vi "AP2_photoelectron_image_aquisition.vi"() -> ()   [LabVIEW 2023]
panel:
  in  "Tuning Spline Path":path
  in  "Tab Control 2":enum32{"Image Slice"}(tab)
  out "Image Slice":dbl[](graph)
  in  "Calc R pixel":bool
  in  "Center Y":dbl=555.0
  in  "Center X":dbl=548.0
  in  "Tab Control":T1(tab)
  out "B Counts/5F":dbl
  out "Avg Counts/F":dbl
  out "A Counts":u32
  out "B Counts":u32
  out "Total Counts":u32
  out "A Counts/5F":dbl
  in  "Stop Control":bool
  in  "Save Image Button":bool
  in  "Discard Image Button":bool
  in  "Threshold range":cluster{"Lower value":sgl, "Upper value":sgl}={"Lower value"=6.0, "Upper value"=1024.0}
  in  "Region of interest":i32[](array[numeric])
  in  "Number of buffers":u32
  in  "Frame timeout (ms)":u32=1000
  in  "Update img":bool
  out "FPS":dbl
  out "Processing time / ms":u32
  in  "Frequency Doubled":bool
  out "Current Wavelength":dbl
  in  "Wavelength":dbl
  out "Accumulated Image":i16[][](graph)
  # "Monitoring"
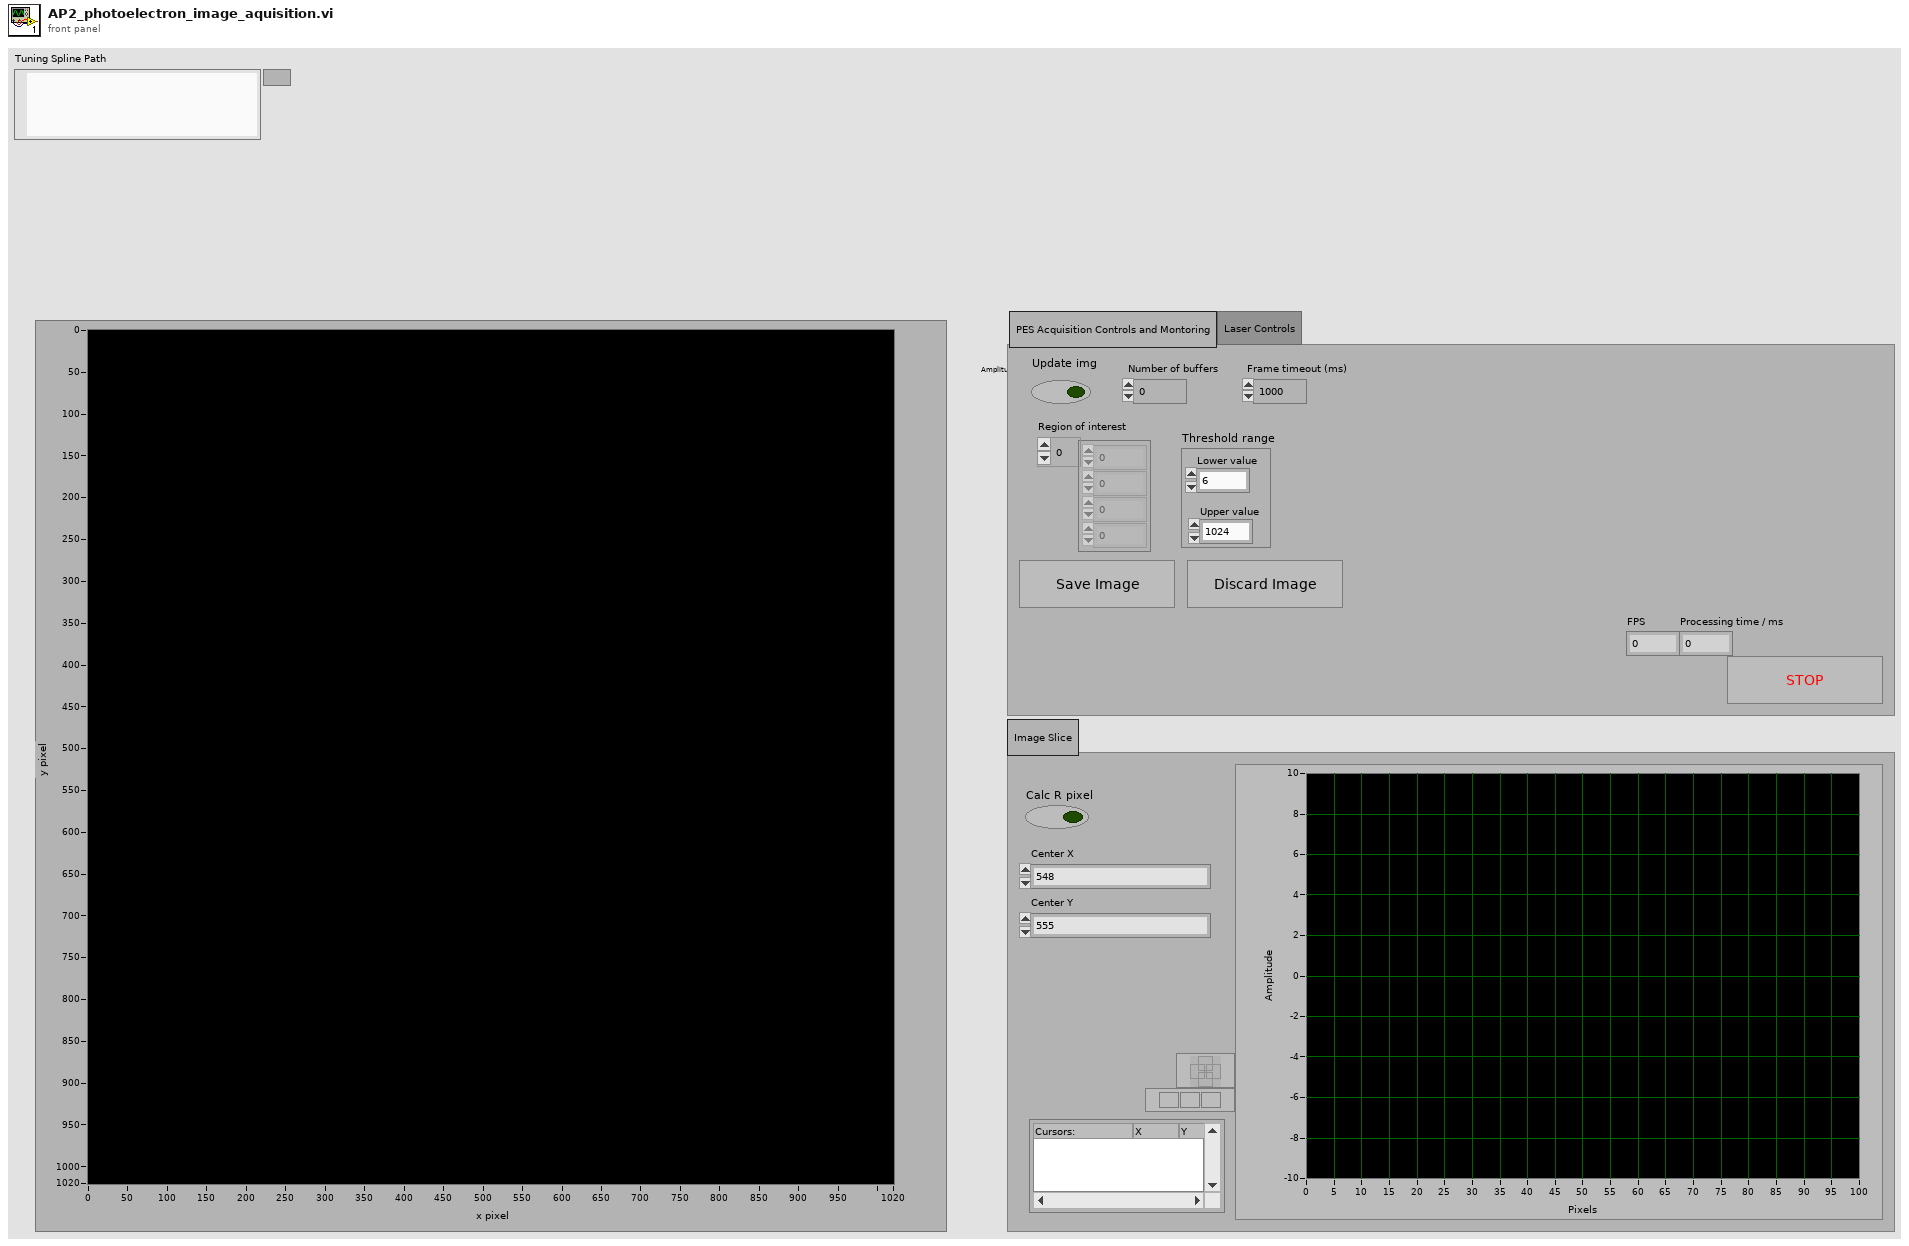
[diagram p1: front panel]
types:
  T1 = enum32{"PES Acquisition Controls and Montoring", "Laser Controls"}
  T2 = cluster{"Region of interest":i32[], "Number of buffers":u32, "Frame timeout (ms)":u32}
  T3 = cluster{"queue out":refnum<queue>, "error out":errorcluster}
  T4 = cluster{"notifier out":refnum<notifier>, "error out":errorcluster}
  T5 = cluster{"i01 data":sgl[][], "i02 data":sgl[][], "Count Buffer Size Out":i32, "Empty Image":i16[][], "Accumulated Image":i16[][], "Corrected Image 1":i16[][], "Corrected Image 2":i16[][], "Total counts":i32, "t_1":i32, "t_2":i32, "t_3":i32, "t_4":i32, "t_5":i32, "t_6":i32, "t_7":i32, "t_8":i32, "t_9":i32, "t_10":i32, "c_1":i32, "c_2":i32, "Region of interest":i32[]}
  T6 = cluster{"Total Counts":u32, "Avg Counts/F":dbl, "B Counts":u32, "A Counts":u32, "A Counts/5F":dbl, "B Counts/5F":dbl}
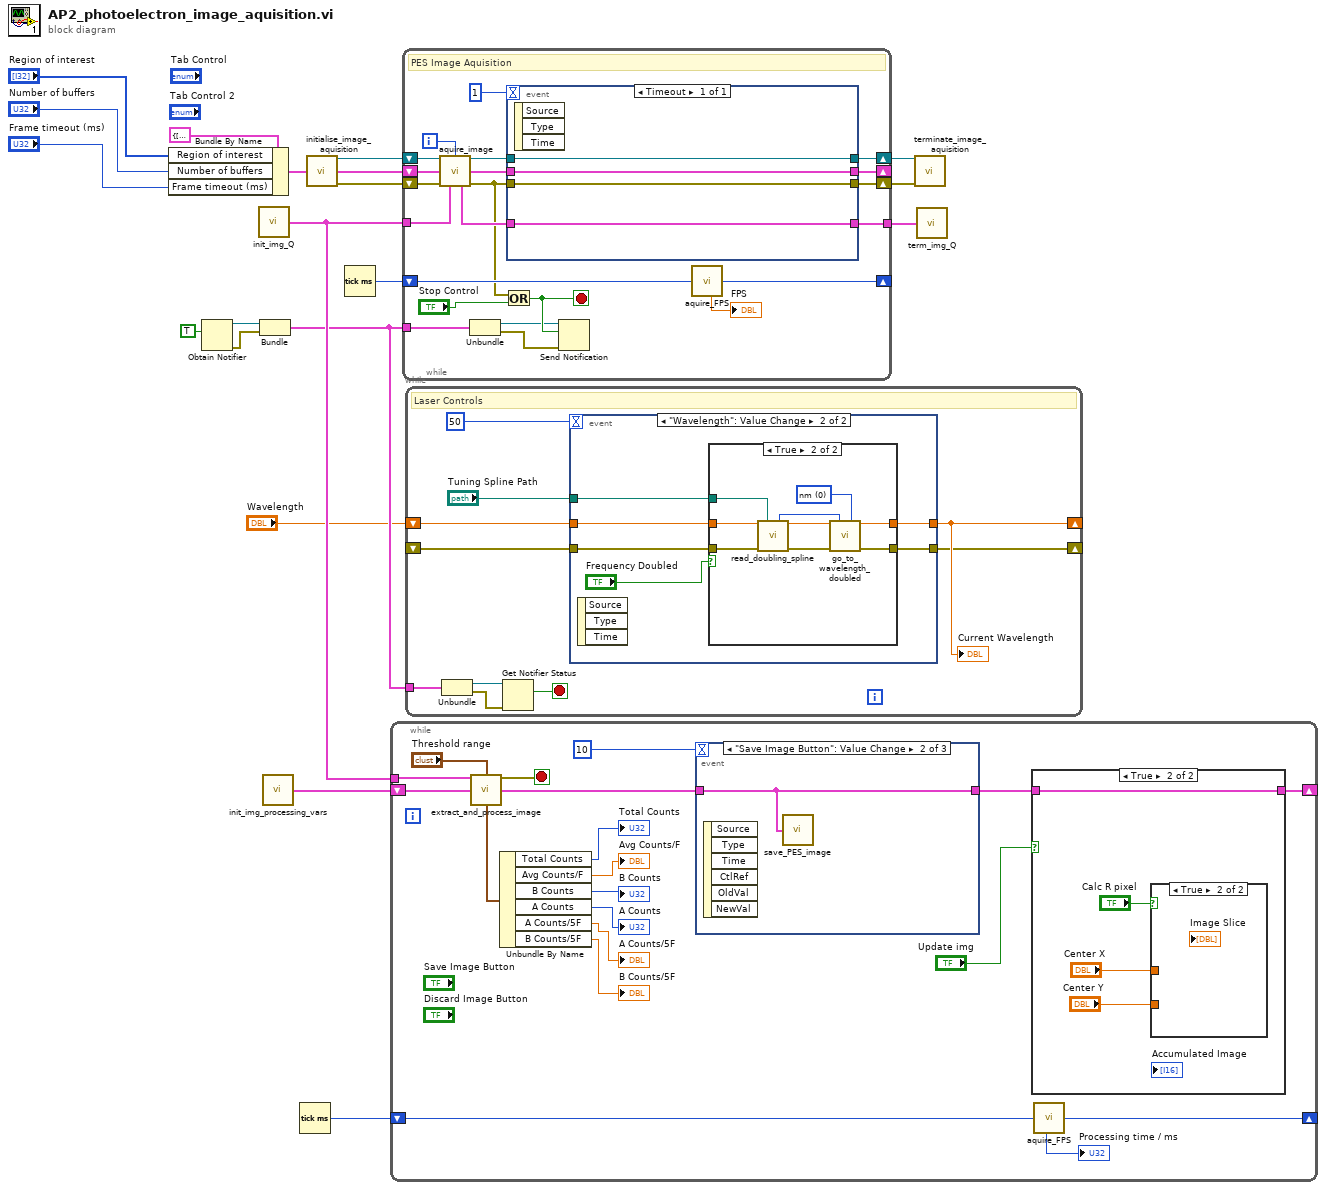
[diagram p0: block diagram]
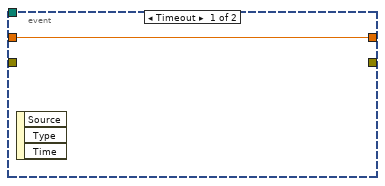
[diagram p2: hidden frame]
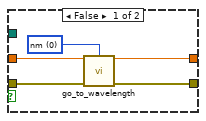
[diagram p3: hidden frame]
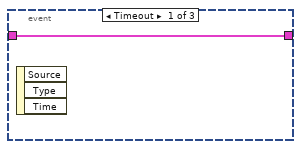
[diagram p4: hidden frame]
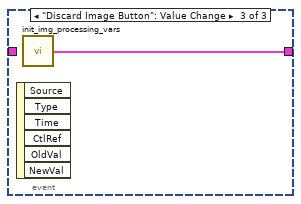
[diagram p5: hidden frame]
diagram:
  n1 = Bundle By Name(cluster=T2 {"Region of interest"=[], "Number of buffers"=0, "Frame timeout (ms)"=1000}, "Region of interest"="Region of interest", "Number of buffers"="Number of buffers", "Frame timeout (ms)"="Frame timeout (ms)") -> (w14:T2)
  n2 = Obtain Notifier(notification data type=TRUE) -> (notifier out=w4:refnum<notifier>, error out=w3:errorcluster)  [unwired: 3 in, 1 out]
  n3 = call "init_img_Q.vi"() -> ("Image Q Out"=w11:T3)  [unwired: 15 in]
  n4 = Bundle("notifier out"=w4, "error out"=w3) -> (w2:T4)  [unwired: 1 in]
  n5 = call "init_img_processing_vars.vi"() -> ("Image Processing Data"=w7:T5)  [unwired: 15 in]
  n6 = Tick Count (ms)() -> (millisecond timer value=w8:u32)
  n7 = call "initialise_image_aquisition.vi"("Imaging Variables In"=w14) -> ("IMAQ Session Out"=w20:refnum<k11>, "Imaging Variables Out"=w13:T2, "error out"=w19:errorcluster)  [unwired: 11 in, 1 out]
  n8 = Tick Count (ms)() -> (millisecond timer value=w6:u32)
  n9 = while {
    tunnel: w11 -> [w36]
    shift-right: [w37] -> _
    shift-left: w8 -> [w38]
    shift-right: [w33] -> _
    shift-left: w7 -> [w34]
    stop <- w35 stop-if-true
    n10 = call "extract_and_process_image.vi"("Image Q In"=w36, "Threshold range"="Threshold range", "Processed Image Data In"=w34) -> ("error out"=w35:errorcluster, "Processed Image Data Out"=w31:T5, "Count data"=w28:T6)  [unwired: 10 in]
    n11 = Unbundle By Name(w28) -> ("Total Counts"=→"Total Counts":u32, "Avg Counts/F"=→"Avg Counts/F":dbl, "B Counts"=→"B Counts":u32, "A Counts"=→"A Counts":u32, "A Counts/5F"=→"A Counts/5F":dbl, "B Counts/5F"=→"B Counts/5F":dbl)
    n12 = event shown="[1] \"Save Image Button\": Value Change" {
      selector: _ -> [_ _ _]
      dyn-events: _ -> [_ _ _]
      timeout: 10 -> [_ _ _]
      tunnel: w31 -> [w40 w41 _]
      tunnel: [w40 w41 w42] -> w29
      event Timeout {
        n13 = event-data() -> ()  [unwired: 1 in, 3 out]
      }
      event "Save Image Button": Value Change {
        n14 = event-data() -> ()  [unwired: 1 in, 6 out]
        n15 = call "save_PES_image.vi"("Processed Image Data In"=w41) -> ()  [unwired: 15 in]
      }
      event "Discard Image Button": Value Change {
        n16 = event-data() -> ()  [unwired: 1 in, 6 out]
        n17 = call "init_img_processing_vars.vi"() -> ("Image Processing Data"=w42:T5)  [unwired: 15 in]
      }
    }
    n18 = case shown="True" "Update img" {
      tunnel: w29 -> [w43 w44]
      tunnel: [w43 w44] -> w33
      frame False {
      }
      frame True {
        n19 = case shown="True" "Calc R pixel" {
          tunnel: "Center X" -> [_ _]
          tunnel: "Center Y" -> [_ _]
          frame False {
          }
          frame True {
          }
        }
      }
    }
    n20 = call "aquire_FPS.vi"("Time Value In /ms"=w38) -> ("Time Value Out /ms"=w37:u32, "Execution time / ms"=→"Processing time / ms":u32)  [unwired: 12 in, 1 out]
  }
  n21 = while {
    shift-right: [w68] -> w10
    shift-left: w20 -> [w65]
    shift-right: [w66] -> w9
    shift-left: w19 -> [w64]
    tunnel: w11 -> [w58]
    tunnel: [w57] -> w12
    shift-right: [w67] -> _
    shift-left: w13 -> [w61]
    shift-right: [w54] -> _
    shift-left: w6 -> [w56]
    tunnel: w2 -> [w50]
    i -> [w63]
    stop <- w51 stop-if-true
    # "PES Image Aquisition"
    n22 = call "aquire_image.vi"("IMAQ Session In"=w65, "Buffer to extract"=w63, "Imaging Variables In"=w61, "error in (no error)"=w64, "Img Q Data In"=w58) -> ("IMAQ Session Out"=w62:refnum<k11>, "Imaging Variables Out"=w60:T2, "Img Q Data Out"=w59:T3, "error out"=w53:errorcluster)  [unwired: 7 in]
    n23 = Unbundle(w50) -> ("notifier out"=w48:refnum<notifier>, "error out"=w49:errorcluster)
    n24 = Or(x=w53, y="Stop Control") -> (x .or. y?=w51:bool)
    n25 = event shown="[0] Timeout" {
      selector: _ -> [_]
      dyn-events: _ -> [_]
      timeout: 1 -> [_]
      tunnel: w62 -> [w73]
      tunnel: w53 -> [w72]
      tunnel: [w73] -> w68
      tunnel: [w72] -> w66
      tunnel: w60 -> [w71]
      tunnel: [w71] -> w67
      tunnel: w59 -> [w70]
      tunnel: [w70] -> w57
      event Timeout {
        n26 = event-data() -> ()  [unwired: 1 in, 3 out]
      }
    }
    n27 = Send Notification(notification=w51, notifier=w48, error in (no error)=w49) -> ()  [unwired: 2 out]
    n28 = call "aquire_FPS.vi"("Time Value In /ms"=w56) -> ("Time Value Out /ms"=w54:u32, "FPS"=→"FPS":dbl)  [unwired: 12 in, 1 out]
  }
  n29 = while {
    tunnel: w2 -> [w83]
    shift-right: [w77] -> _
    shift-left: "Wavelength" -> [w78]
    shift-right: [w76] -> _
    shift-left: _ -> [w75]
    stop <- w80 stop-if-true
    # "Laser Controls"
    n30 = Unbundle(w83) -> ("notifier out"=w82:refnum<notifier>, "error out"=w81:errorcluster)
    n31 = Get Notifier Status(notifier=w82, error in (no error)=w81) -> (current notification=w80:bool)  [unwired: 4 out]
    n32 = event shown="[1] \"Wavelength\": Value Change" {
      selector: _ -> [_ _]
      dyn-events: _ -> [_ _]
      timeout: 50 -> [_ _]
      tunnel: w78 -> [w84 w89]
      tunnel: [w84 w88] -> w77
      tunnel: [_ w87] -> w76
      tunnel: w75 -> [_ w86]
      tunnel: "Tuning Spline Path" -> [_ w85]
      event Timeout {
        n33 = event-data() -> ()  [unwired: 1 in, 3 out]
      }
      event "Wavelength": Value Change {
        n34 = event-data() -> ()  [unwired: 1 in, 3 out]
        n35 = case shown="True" "Frequency Doubled" {
          tunnel: w89 -> [w95 w102]
          tunnel: [w94 w104] -> w88
          tunnel: [w93 w103] -> w87
          tunnel: w86 -> [w92 w101]
          tunnel: w85 -> [_ w97]
          frame False {
            w91 = u16 0 items=["nm", "cm-1"] ("Unit")
            n36 = call "go_to_wavelength.vi"("Set Laser Position"=w95, "Unit"=w91, "error in (no error)"=w92) -> ("Current Laser Position"=w94:dbl, "error out"=w93:errorcluster)  [unwired: 11 in]
          }
          frame True {
            w96 = u16 0 items=["nm", "cm-1"] ("Unit")
            n37 = call "read_doubling_spline.vi"("Wavelength"=w102, "Tuning Spline Path"=w97, "Error In"=w101) -> ("BBO Position"=w98:i32, "Wavelength Out"=w99:dbl, "Error Out"=w100:errorcluster)  [unwired: 10 in]
            n38 = call "go_to_wavelength_doubled.vi"("Set Laser Position"=w99, "Set BBO crystal position"=w98, "Unit"=w96, "error in (no error)"=w100) -> ("Current Laser Position"=w104:dbl, "error out"=w103:errorcluster)  [unwired: 10 in]
          }
        }
      }
    }
    "Current Wavelength" <- w77
  }
  n39 = call "terminate_image_aquisition.vi"("IMAQ Session In"=w10, "error in (no error)"=w9) -> ()  [unwired: 13 in, 1 out]
  n40 = call "term_img_Q.vi"("Image Q Out"=w12) -> ()  [unwired: 14 in, 1 out]
